vi "CreateMonitor.vi"(11 "File Path Control":path) -> (0 "error out":errorcluster, 3 "Handle":i32)   [LabVIEW 2016]
uses:
  kernel32.dll
panel:
  in  "error in":errorcluster
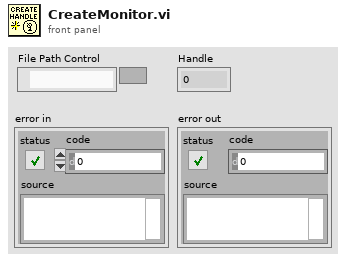
[diagram p1: front panel]
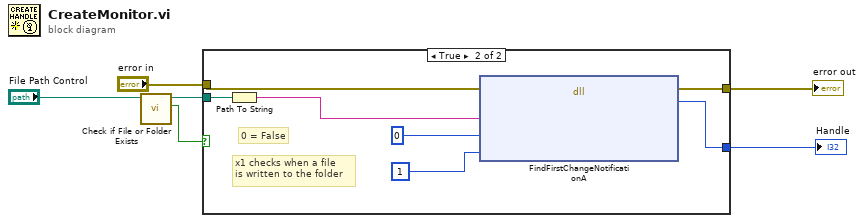
[diagram p0: block diagram]
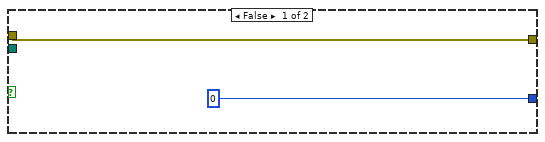
[diagram p2: hidden frame]
diagram:
  n1 = call <vilib>:"Check if File or Folder Exists.vi"("path"="File Path Control") -> ("file or folder exists?"=w2:bool, "dup path"=w1:path)  [unwired: 8 in, 1 out]
  n2 = case shown="True" w2 {
    tunnel: [0 ("Handle") w15] -> w6
    tunnel: [w7 w14] -> w5
    tunnel: "error in" -> [w7 w10]
    tunnel: w1 -> [_ w9]
    frame False {
    }
    frame True {
      # "0 = False"
      # "x1 checks when a file\nis written to the folder"
      n3 = Path To String(path=w9) -> (string=w11:string)
      n4 = dll-call lib="kernel32.dll" fn="FindFirstChangeNotificationA"(error in=w10, "pathName"=w11, "watchSubtree"=u8 0, "NotifyFilter"=u32 1) -> (error out=w14:errorcluster, "Handle"=w15:i32)  [unwired: 5 in, 1 out]
    }
  }
  "Handle" <- w6
  "error out" <- w5
